vi "get structure diagram.vi"(8 "error in":errorcluster, 10 "index":i32, 11 "structure_id":string) -> (0 "error out":errorcluster, 3 "diagram_id":string)   [LabVIEW 2020]
doc: "Returns a reference to a subdiagram of a structure (loop, case structure etc.) defined by index. Use index 0 for loops, only use index > 0 for multi-frame structures."
uses:
  G-AI Core/G-AI Core.lvlib
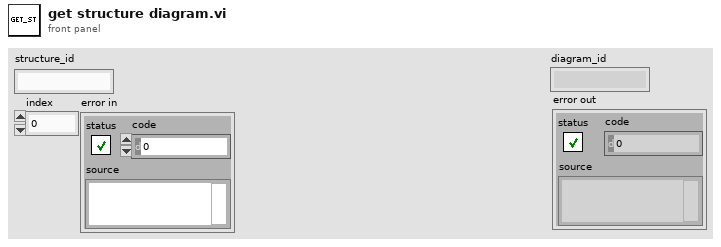
[diagram p1: front panel]
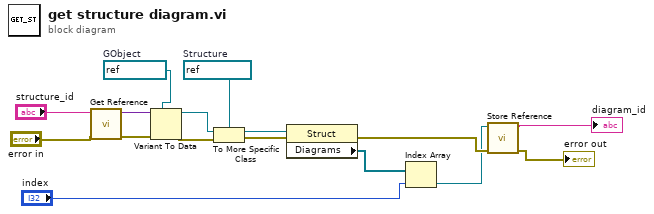
[diagram p0: block diagram]
diagram:
  w11 = refnum<vi> refnum  # GObject
  w12 = refnum<vi> refnum  # Structure
  n1 = call "Get Reference.vi"("error in"="error in", "id"="structure_id") -> ("error out"=w15:errorcluster, "reference"=w14:variant)  [unwired: 8 in]
  n2 = Variant To Data(error in=w15, type=w11, Variant=w14) -> (data=w10:refnum<vi>, error out=w13:errorcluster)
  n3 = To More Specific Class(target class=w12, reference=w10, error in=w13) -> (specific class reference=w8:refnum<vi>, error out=w9:errorcluster)
  n4 = property class="Struct"(reference=w8, error in=w9) -> (error out=w6:errorcluster, "Diagrams"=w7:refnum<vi>[])  [unwired: 1 out]
  n5 = Index Array(array=w7, index="index") -> (element=w5:refnum<vi>)
  n6 = call "Store Reference.vi"("error in"=w6, "Reference"=w5) -> ("error out"=→"error out":errorcluster, "id"=→"diagram_id":string)  [unwired: 8 in]
